vi "Configure Waveform (Staircase).vi"(0 "VISA resource name":refnum<visa-resource-name>, 1 "Staircase Start Time (0.0 s)":dbl format="%^.3e", 2 "Staircase Start Level (0.0)":dbl format="%^.3e", 3 "Staircase Total Time (1.0 s)":dbl=1.0 format="%^.3e", 5 "Channel Name (1)":string="1", 7 "Staircase Steps (10)":i32=10, 9 "Waveform Type (1: Voltage)":i32(ring)=1 items=["Voltage"=1, "Current"=0], 11 "error in (no error)":errorcluster {"code" format="%.0x"}, 12 "Staircase End Time (0.0 s)":dbl format="%^.3e", 13 "Staircase End Level (0.0)":dbl format="%^.3e") -> (4 "VISA resource name out":refnum<visa-resource-name>, 15 "error out":errorcluster {"code" format="%.0x"})   [LabVIEW 2018, in "Agilent N6700 Series.lvlib"]
doc: "Configures the staircase waveform.\n\n<b>Note:</b>\nThis VI only applies to the N6705B and N6705C DC Power Analyzer."
uses:
  Agilent N6700 Series.lvlib
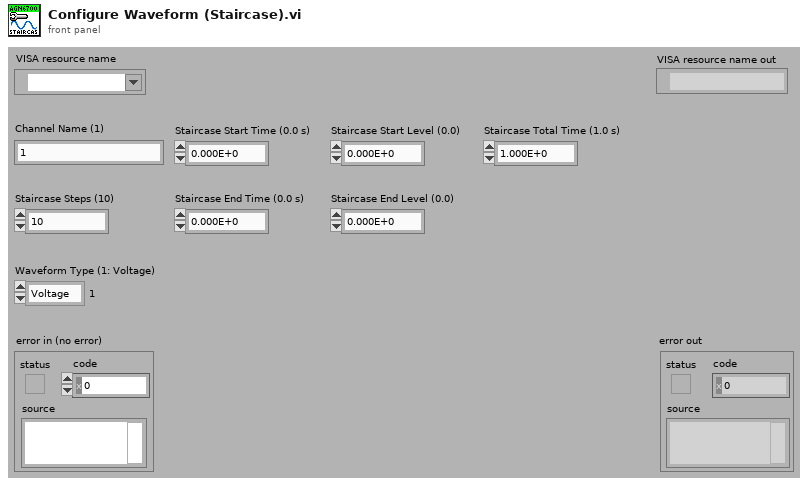
[diagram p1: front panel]
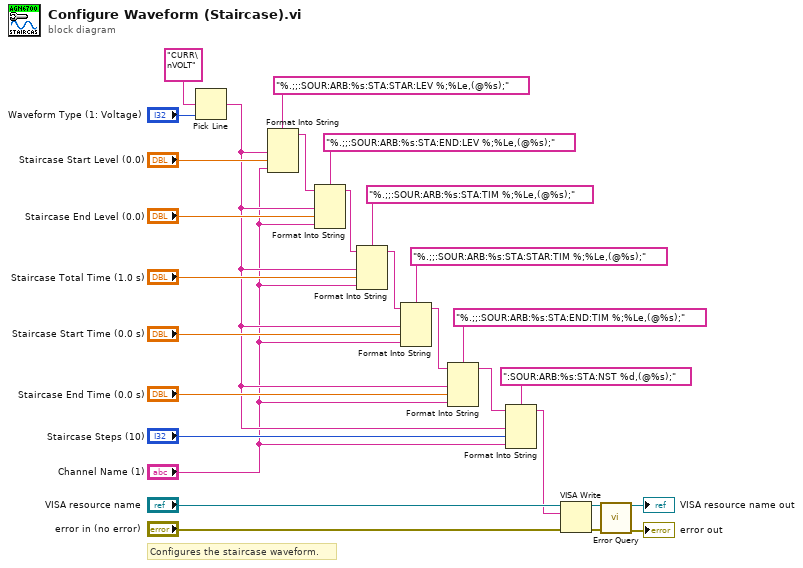
[diagram p0: block diagram]
diagram:
  # "Configures the staircase waveform."
  n1 = Pick Line(multi-line string="CURR\nVOLT", line index="Waveform Type (1: Voltage)") -> (output string=w2:string)  [unwired: 1 in]
  n2 = Format Into String(format string="%.;;:SOUR:ARB:%s:STA:STAR:LEV %;%Le,(@%s);", w2, "Staircase Start Level (0.0)", "Channel Name (1)") -> (resulting string=w18:string)  [unwired: 2 in, 1 out]
  n3 = Format Into String(format string="%.;;:SOUR:ARB:%s:STA:END:LEV %;%Le,(@%s);", initial string=w18, w2, "Staircase End Level (0.0)", "Channel Name (1)") -> (resulting string=w17:string)  [unwired: 1 in, 1 out]
  n4 = Format Into String(format string="%.;;:SOUR:ARB:%s:STA:TIM %;%Le,(@%s);", initial string=w17, w2, "Staircase Total Time (1.0 s)", "Channel Name (1)") -> (resulting string=w16:string)  [unwired: 1 in, 1 out]
  n5 = Format Into String(format string="%.;;:SOUR:ARB:%s:STA:STAR:TIM %;%Le,(@%s);", initial string=w16, w2, "Staircase Start Time (0.0 s)", "Channel Name (1)") -> (resulting string=w15:string)  [unwired: 1 in, 1 out]
  n6 = Format Into String(format string="%.;;:SOUR:ARB:%s:STA:END:TIM %;%Le,(@%s);", initial string=w15, w2, "Staircase End Time (0.0 s)", "Channel Name (1)") -> (resulting string=w5:string)  [unwired: 1 in, 1 out]
  n7 = Format Into String(format string=":SOUR:ARB:%s:STA:NST %d,(@%s);", initial string=w5, w2, "Staircase Steps (10)", "Channel Name (1)") -> (resulting string=w3:string)  [unwired: 1 in, 1 out]
  n8 = VISA Write(VISA resource name="VISA resource name", write buffer=w3, error in (no error)="error in (no error)") -> (VISA resource name out=w24:refnum<visa-resource-name>, error out=w23:errorcluster)  [unwired: 1 out]
  n9 = call "Error Query.vi"("VISA resource name"=w24, "error in (no error)"=w23) -> ("VISA resource name out"=→"VISA resource name out":refnum<visa-resource-name>, "error out"=→"error out":errorcluster)  [unwired: 10 in, 2 out]
